vi "输入数据解析.vi"(0 "单个参数补充":dbl, 1 "从板号":dbl=1.0, 2 "主板二维码":string="BNET01", 3 "从板二维码":string="BNET01", 5 "主板引用":refnum<vi>, 7 "从板引用":refnum<vi>, 9 "主板选项":string="三级故障阀值", 11 "枚举":enum16{"主板", "从板"}(ring), 12 "快换":bool caption="快换写入") -> (4 "输出数组":dbl[][](array[numeric]), 6 "数组长度":dbl[](array[numeric]), 8 "循环次数":i32, 10 "命令":u32, 14 "名称":string[](array[string]), 15 "命令序号":u32[](array[numeric]))   [LabVIEW 2013] (continued)
              tunnel: [w13384 w13395 w13406 w13418 w13429 w13440 w13452 w13462] -> w13379
              frame 0, Default {
                # "最大允许单体电压"
                n5117 = disable-structure shown="启用" {
                  disable-tunnel: [w13390 w13393] -> w13386
                  disable-tunnel: [w13389 w13393] -> w13385
                  disable-tunnel: w13383 -> [w13388 _]
                  frame Disabled {
                    n5118 = Unbundle By Name(w13388) -> ("最大允许单体电压"=w13387:dbl)
                    n5119 = call "输入分辨率计算-EV05.vi"("1字节?"=FALSE, "数值"=w13387, "分辨率"=0.001) -> ("低字节"=w13389:dbl, "高字节1"=w13390:dbl)  [unwired: 2 in, 5 out]
                  }
                  frame Enabled {
                    w13393 = 255 ("高字节1")
                  }
                }
                n5120 = Build Array(w13386, w13385) -> (w13384:i32[])
              }
              frame 1 {
                # "最大允许总电压"
                n5121 = disable-structure shown="启用" {
                  disable-tunnel: [w13401 w13404] -> w13397
                  disable-tunnel: [w13400 w13404] -> w13396
                  disable-tunnel: w13394 -> [w13399 _]
                  frame Disabled {
                    n5122 = Unbundle By Name(w13399) -> ("最大允许总电压"=w13398:dbl)
                    n5123 = call "输入分辨率计算-EV05.vi"("1字节?"=FALSE, "数值"=w13398, "分辨率"=0.1) -> ("低字节"=w13400:dbl, "高字节1"=w13401:dbl)  [unwired: 2 in, 5 out]
                  }
                  frame Enabled {
                    w13404 = 255 ("高字节1")
                  }
                }
                n5124 = Build Array(w13397, w13396) -> (w13395:i32[])
              }
              frame 2 {
                # "最大允许充电电流"
                n5125 = disable-structure shown="启用" {
                  disable-tunnel: [w13413 w13416] -> w13408
                  disable-tunnel: [w13412 w13416] -> w13407
                  disable-tunnel: w13405 -> [w13410 _]
                  frame Enabled {
                    n5126 = Unbundle By Name(w13410) -> ("最大允许充电电流"=w13409:dbl)
                    n5127 = call "输入分辨率计算-EV05.vi"("1字节?"=FALSE, "数值"=w13409, "偏移量"=0.0, "分辨率"=0.1) -> ("低字节"=w13412:dbl, "高字节1"=w13413:dbl)  [unwired: 1 in, 5 out]
                  }
                  frame Disabled {
                    w13416 = 255 ("高字节1")
                  }
                }
                n5128 = Build Array(w13408, w13407) -> (w13406:dbl[])
              }
              frame 3 {
                # "最小允许充电温度"
                n5129 = disable-structure shown="启用" {
                  disable-tunnel: [w13423 255 ("高字节1")] -> w13419
                  disable-tunnel: w13417 -> [w13421 _]
                  frame Disabled {
                    n5130 = Unbundle By Name(w13421) -> ("最小允许温度"=w13420:dbl)
                    n5131 = call "输入分辨率计算-EV05.vi"("1字节?"=TRUE, "数值"=w13420, "偏移量"=-40.0, "分辨率"=1.0) -> ("高字节1"=w13423:dbl)  [unwired: 1 in, 6 out]
                  }
                  frame Enabled {
                  }
                }
                n5132 = Build Array(w13419) -> (w13418:i32[])
              }
              frame 4 {
                # "最小充电电流"
                n5133 = disable-structure shown="启用" {
                  disable-tunnel: [w13434 w13437] -> w13430
                  disable-tunnel: [w13433 w13437] -> w13428
                  disable-tunnel: w13427 -> [w13432 _]
                  frame Disabled {
                    n5134 = Unbundle By Name(w13432) -> ("最小充电电流"=w13431:dbl)
                    n5135 = call "输入分辨率计算-EV05.vi"("1字节?"=FALSE, "数值"=w13431, "分辨率"=0.1) -> ("低字节"=w13433:dbl, "高字节1"=w13434:dbl)  [unwired: 2 in, 5 out]
                  }
                  frame Enabled {
                    w13437 = 255 ("高字节1")
                  }
                }
                n5136 = Build Array(w13430, w13428) -> (w13429:i32[])
              }
              frame 5 {
                # "电流步长"
                n5137 = disable-structure shown="启用" {
                  disable-tunnel: [w13446 w13449] -> w13441
                  disable-tunnel: [w13444 w13449] -> w13439
                  disable-tunnel: w13438 -> [w13443 _]
                  frame Disabled {
                    n5138 = Unbundle By Name(w13443) -> ("电流步长"=w13442:dbl)
                    n5139 = call "输入分辨率计算-EV05.vi"("1字节?"=FALSE, "数值"=w13442, "偏移量"=0.0, "分辨率"=1.0) -> ("低字节"=w13444:dbl, "高字节1"=w13446:dbl)  [unwired: 1 in, 5 out]
                  }
                  frame Enabled {
                    w13449 = 255 ("高字节1")
                  }
                }
                n5140 = Build Array(w13441, w13439) -> (w13440:i32[])
              }
              frame 6 {
                # "最小允许单体电压"
                n5141 = disable-structure shown="启用" {
                  disable-tunnel: [w13457 w13460] -> w13453
                  disable-tunnel: [w13456 w13460] -> w13451
                  disable-tunnel: w13450 -> [w13455 _]
                  frame Disabled {
                    n5142 = Unbundle By Name(w13455) -> ("最小允许单体电压"=w13454:dbl)
                    n5143 = call "输入分辨率计算-EV05.vi"("1字节?"=FALSE, "数值"=w13454, "分辨率"=0.001) -> ("低字节"=w13456:dbl, "高字节1"=w13457:dbl)  [unwired: 2 in, 5 out]
                  }
                  frame Enabled {
                    w13460 = 255 ("高字节1")
                  }
                }
                n5144 = Build Array(w13453, w13451) -> (w13452:i32[])
              }
              frame 7 {
                # "最大允许充电温度"
                n5145 = disable-structure shown="启用" {
                  disable-tunnel: [w13467 255 ("高字节1")] -> w13463
                  disable-tunnel: w13461 -> [w13465 _]
                  frame Disabled {
                    n5146 = Unbundle By Name(w13465) -> ("最大允许充电温度"=w13464:dbl)
                    n5147 = call "输入分辨率计算-EV05.vi"("1字节?"=TRUE, "数值"=w13464, "偏移量"=-40.0, "分辨率"=1.0) -> ("高字节1"=w13467:dbl)  [unwired: 1 in, 6 out]
                  }
                  frame Enabled {
                  }
                }
                n5148 = Build Array(w13463) -> (w13462:i32[])
              }
            }
            n5149 = Insert Into Array(array=w13378, new element=w13379) -> (w13382:dbl[])  [unwired: 1 in]
          }
          n5150 = Build Array(w13374) -> (w13376:dbl[][])
        }
        frame "最小允许充电温度" {
          n5151 = Unbundle By Name(w13474) -> ("充电控制参数"=w13475:refnum<vi>)
          n5152 = property class="Clust (严格)"(reference=w13475) -> ("Value"=w13473:T6)  [unwired: 1 in, 2 out]
          n5153 = for {
            N: 8 -> [_]
            tunnel: w13473 -> [w13485]
            shift-right: [w13487] -> w13479
            shift-left: dbl[] [] -> [w13483]
            i -> [w13486]
            n5154 = case shown="3" w13486 {
              tunnel: w13485 -> [w13488 w13499 w13510 w13522 w13532 w13543 w13555 w13566]
              tunnel: [w13489 w13500 w13511 w13523 w13534 w13545 w13557 w13567] -> w13484
              frame 0, Default {
                # "最大允许单体电压"
                n5155 = disable-structure shown="启用" {
                  disable-tunnel: [w13495 w13498] -> w13491
                  disable-tunnel: [w13494 w13498] -> w13490
                  disable-tunnel: w13488 -> [w13493 _]
                  frame Disabled {
                    n5156 = Unbundle By Name(w13493) -> ("最大允许单体电压"=w13492:dbl)
                    n5157 = call "输入分辨率计算-EV05.vi"("1字节?"=FALSE, "数值"=w13492, "分辨率"=0.001) -> ("低字节"=w13494:dbl, "高字节1"=w13495:dbl)  [unwired: 2 in, 5 out]
                  }
                  frame Enabled {
                    w13498 = 255 ("高字节1")
                  }
                }
                n5158 = Build Array(w13491, w13490) -> (w13489:i32[])
              }
              frame 1 {
                # "最大允许总电压"
                n5159 = disable-structure shown="启用" {
                  disable-tunnel: [w13506 w13509] -> w13502
                  disable-tunnel: [w13505 w13509] -> w13501
                  disable-tunnel: w13499 -> [w13504 _]
                  frame Disabled {
                    n5160 = Unbundle By Name(w13504) -> ("最大允许总电压"=w13503:dbl)
                    n5161 = call "输入分辨率计算-EV05.vi"("1字节?"=FALSE, "数值"=w13503, "分辨率"=0.1) -> ("低字节"=w13505:dbl, "高字节1"=w13506:dbl)  [unwired: 2 in, 5 out]
                  }
                  frame Enabled {
                    w13509 = 255 ("高字节1")
                  }
                }
                n5162 = Build Array(w13502, w13501) -> (w13500:i32[])
              }
              frame 2 {
                # "最大允许充电电流"
                n5163 = disable-structure shown="启用" {
                  disable-tunnel: [w13518 w13521] -> w13513
                  disable-tunnel: [w13517 w13521] -> w13512
                  disable-tunnel: w13510 -> [w13515 _]
                  frame Disabled {
                    n5164 = Unbundle By Name(w13515) -> ("最大允许充电电流"=w13514:dbl)
                    n5165 = call "输入分辨率计算-EV05.vi"("1字节?"=FALSE, "数值"=w13514, "偏移量"=-3000.0, "分辨率"=0.1) -> ("低字节"=w13517:dbl, "高字节1"=w13518:dbl)  [unwired: 1 in, 5 out]
                  }
                  frame Enabled {
                    w13521 = 255 ("高字节1")
                  }
                }
                n5166 = Build Array(w13513, w13512) -> (w13511:i32[])
              }
              frame 3 {
                # "最小允许充电温度"
                n5167 = disable-structure shown="启用" {
                  disable-tunnel: [w13528 255 ("高字节1")] -> w13524
                  disable-tunnel: w13522 -> [w13526 _]
                  frame Enabled {
                    n5168 = Unbundle By Name(w13526) -> ("最小允许充电温度"=w13525:dbl)
                    n5169 = call "输入分辨率计算-EV05.vi"("1字节?"=TRUE, "数值"=w13525, "偏移量"=-40.0, "分辨率"=1.0) -> ("高字节1"=w13528:dbl)  [unwired: 1 in, 6 out]
                  }
                  frame Disabled {
                  }
                }
                n5170 = Build Array(w13524) -> (w13523:dbl[])
              }
              frame 4 {
                # "最小充电电流"
                n5171 = disable-structure shown="启用" {
                  disable-tunnel: [w13539 w13542] -> w13535
                  disable-tunnel: [w13538 w13542] -> w13533
                  disable-tunnel: w13532 -> [w13537 _]
                  frame Disabled {
                    n5172 = Unbundle By Name(w13537) -> ("最小充电电流"=w13536:dbl)
                    n5173 = call "输入分辨率计算-EV05.vi"("1字节?"=FALSE, "数值"=w13536, "分辨率"=0.1) -> ("低字节"=w13538:dbl, "高字节1"=w13539:dbl)  [unwired: 2 in, 5 out]
                  }
                  frame Enabled {
                    w13542 = 255 ("高字节1")
                  }
                }
                n5174 = Build Array(w13535, w13533) -> (w13534:i32[])
              }
              frame 5 {
                # "电流步长"
                n5175 = disable-structure shown="启用" {
                  disable-tunnel: [w13551 w13554] -> w13546
                  disable-tunnel: [w13549 w13554] -> w13544
                  disable-tunnel: w13543 -> [w13548 _]
                  frame Disabled {
                    n5176 = Unbundle By Name(w13548) -> ("电流步长"=w13547:dbl)
                    n5177 = call "输入分辨率计算-EV05.vi"("1字节?"=FALSE, "数值"=w13547, "偏移量"=0.0, "分辨率"=1.0) -> ("低字节"=w13549:dbl, "高字节1"=w13551:dbl)  [unwired: 1 in, 5 out]
                  }
                  frame Enabled {
                    w13554 = 255 ("高字节1")
                  }
                }
                n5178 = Build Array(w13546, w13544) -> (w13545:i32[])
              }
              frame 6 {
                # "最小允许单体电压"
                n5179 = disable-structure shown="启用" {
                  disable-tunnel: [w13562 w13565] -> w13558
                  disable-tunnel: [w13561 w13565] -> w13556
                  disable-tunnel: w13555 -> [w13560 _]
                  frame Disabled {
                    n5180 = Unbundle By Name(w13560) -> ("最小允许单体电压"=w13559:dbl)
                    n5181 = call "输入分辨率计算-EV05.vi"("1字节?"=FALSE, "数值"=w13559, "分辨率"=0.001) -> ("低字节"=w13561:dbl, "高字节1"=w13562:dbl)  [unwired: 2 in, 5 out]
                  }
                  frame Enabled {
                    w13565 = 255 ("高字节1")
                  }
                }
                n5182 = Build Array(w13558, w13556) -> (w13557:i32[])
              }
              frame 7 {
                # "最大允许充电温度"
                n5183 = disable-structure shown="启用" {
                  disable-tunnel: [w13572 255 ("高字节1")] -> w13568
                  disable-tunnel: w13566 -> [w13570 _]
                  frame Disabled {
                    n5184 = Unbundle By Name(w13570) -> ("最大允许充电温度"=w13569:dbl)
                    n5185 = call "输入分辨率计算-EV05.vi"("1字节?"=TRUE, "数值"=w13569, "偏移量"=-40.0, "分辨率"=1.0) -> ("高字节1"=w13572:dbl)  [unwired: 1 in, 6 out]
                  }
                  frame Enabled {
                  }
                }
                n5186 = Build Array(w13568) -> (w13567:i32[])
              }
            }
            n5187 = Insert Into Array(array=w13483, new element=w13484) -> (w13487:dbl[])  [unwired: 1 in]
          }
          n5188 = Build Array(w13479) -> (w13481:dbl[][])
        }
        frame "最小允许充电电流" {
          n5189 = Unbundle By Name(w13579) -> ("充电控制参数"=w13580:refnum<vi>)
          n5190 = property class="Clust (严格)"(reference=w13580) -> ("Value"=w13578:T6)  [unwired: 1 in, 2 out]
          n5191 = for {
            N: 8 -> [_]
            tunnel: w13578 -> [w13590]
            shift-right: [w13592] -> w13584
            shift-left: dbl[] [] -> [w13588]
            i -> [w13591]
            n5192 = case shown="4" w13591 {
              tunnel: w13590 -> [w13593 w13604 w13615 w13627 w13637 w13648 w13660 w13671]
              tunnel: [w13594 w13605 w13616 w13628 w13639 w13650 w13662 w13672] -> w13589
              frame 0, Default {
                # "最大允许单体电压"
                n5193 = disable-structure shown="启用" {
                  disable-tunnel: [w13600 w13603] -> w13596
                  disable-tunnel: [w13599 w13603] -> w13595
                  disable-tunnel: w13593 -> [w13598 _]
                  frame Disabled {
                    n5194 = Unbundle By Name(w13598) -> ("最大允许单体电压"=w13597:dbl)
                    n5195 = call "输入分辨率计算-EV05.vi"("1字节?"=FALSE, "数值"=w13597, "分辨率"=0.001) -> ("低字节"=w13599:dbl, "高字节1"=w13600:dbl)  [unwired: 2 in, 5 out]
                  }
                  frame Enabled {
                    w13603 = 255 ("高字节1")
                  }
                }
                n5196 = Build Array(w13596, w13595) -> (w13594:i32[])
              }
              frame 1 {
                # "最大允许总电压"
                n5197 = disable-structure shown="启用" {
                  disable-tunnel: [w13611 w13614] -> w13607
                  disable-tunnel: [w13610 w13614] -> w13606
                  disable-tunnel: w13604 -> [w13609 _]
                  frame Disabled {
                    n5198 = Unbundle By Name(w13609) -> ("最大允许总电压"=w13608:dbl)
                    n5199 = call "输入分辨率计算-EV05.vi"("1字节?"=FALSE, "数值"=w13608, "分辨率"=0.1) -> ("低字节"=w13610:dbl, "高字节1"=w13611:dbl)  [unwired: 2 in, 5 out]
                  }
                  frame Enabled {
                    w13614 = 255 ("高字节1")
                  }
                }
                n5200 = Build Array(w13607, w13606) -> (w13605:i32[])
              }
              frame 2 {
                # "最大允许充电电流"
                n5201 = disable-structure shown="启用" {
                  disable-tunnel: [w13623 w13626] -> w13618
                  disable-tunnel: [w13622 w13626] -> w13617
                  disable-tunnel: w13615 -> [w13620 _]
                  frame Disabled {
                    n5202 = Unbundle By Name(w13620) -> ("最大允许充电电流"=w13619:dbl)
                    n5203 = call "输入分辨率计算-EV05.vi"("1字节?"=FALSE, "数值"=w13619, "偏移量"=-3000.0, "分辨率"=0.1) -> ("低字节"=w13622:dbl, "高字节1"=w13623:dbl)  [unwired: 1 in, 5 out]
                  }
                  frame Enabled {
                    w13626 = 255 ("高字节1")
                  }
                }
                n5204 = Build Array(w13618, w13617) -> (w13616:i32[])
              }
              frame 3 {
                # "最小允许充电温度"
                n5205 = disable-structure shown="启用" {
                  disable-tunnel: [w13633 255 ("高字节1")] -> w13629
                  disable-tunnel: w13627 -> [w13631 _]
                  frame Disabled {
                    n5206 = Unbundle By Name(w13631) -> ("最小允许温度"=w13630:dbl)
                    n5207 = call "输入分辨率计算-EV05.vi"("1字节?"=TRUE, "数值"=w13630, "偏移量"=-40.0, "分辨率"=1.0) -> ("高字节1"=w13633:dbl)  [unwired: 1 in, 6 out]
                  }
                  frame Enabled {
                  }
                }
                n5208 = Build Array(w13629) -> (w13628:i32[])
              }
              frame 4 {
                # "最小充电电流"
                n5209 = disable-structure shown="启用" {
                  disable-tunnel: [w13644 w13647] -> w13640
                  disable-tunnel: [w13643 w13647] -> w13638
                  disable-tunnel: w13637 -> [w13642 _]
                  frame Enabled {
                    n5210 = Unbundle By Name(w13642) -> ("最小允许充电电流"=w13641:dbl)
                    n5211 = call "输入分辨率计算-EV05.vi"("1字节?"=FALSE, "数值"=w13641, "分辨率"=0.1) -> ("低字节"=w13643:dbl, "高字节1"=w13644:dbl)  [unwired: 2 in, 5 out]
                  }
                  frame Disabled {
                    w13647 = 255 ("高字节1")
                  }
                }
                n5212 = Build Array(w13640, w13638) -> (w13639:dbl[])
              }
              frame 5 {
                # "电流步长"
                n5213 = disable-structure shown="启用" {
                  disable-tunnel: [w13656 w13659] -> w13651
                  disable-tunnel: [w13654 w13659] -> w13649
                  disable-tunnel: w13648 -> [w13653 _]
                  frame Disabled {
                    n5214 = Unbundle By Name(w13653) -> ("电流步长"=w13652:dbl)
                    n5215 = call "输入分辨率计算-EV05.vi"("1字节?"=FALSE, "数值"=w13652, "偏移量"=0.0, "分辨率"=1.0) -> ("低字节"=w13654:dbl, "高字节1"=w13656:dbl)  [unwired: 1 in, 5 out]
                  }
                  frame Enabled {
                    w13659 = 255 ("高字节1")
                  }
                }
                n5216 = Build Array(w13651, w13649) -> (w13650:i32[])
              }
              frame 6 {
                # "最小允许单体电压"
                n5217 = disable-structure shown="启用" {
                  disable-tunnel: [w13667 w13670] -> w13663
                  disable-tunnel: [w13666 w13670] -> w13661
                  disable-tunnel: w13660 -> [w13665 _]
                  frame Disabled {
                    n5218 = Unbundle By Name(w13665) -> ("最小允许单体电压"=w13664:dbl)
                    n5219 = call "输入分辨率计算-EV05.vi"("1字节?"=FALSE, "数值"=w13664, "分辨率"=0.001) -> ("低字节"=w13666:dbl, "高字节1"=w13667:dbl)  [unwired: 2 in, 5 out]
                  }
                  frame Enabled {
                    w13670 = 255 ("高字节1")
                  }
                }
                n5220 = Build Array(w13663, w13661) -> (w13662:i32[])
              }
              frame 7 {
                # "最大允许充电温度"
                n5221 = disable-structure shown="启用" {
                  disable-tunnel: [w13677 255 ("高字节1")] -> w13673
                  disable-tunnel: w13671 -> [w13675 _]
                  frame Disabled {
                    n5222 = Unbundle By Name(w13675) -> ("最大允许充电温度"=w13674:dbl)
                    n5223 = call "输入分辨率计算-EV05.vi"("1字节?"=TRUE, "数值"=w13674, "偏移量"=-40.0, "分辨率"=1.0) -> ("高字节1"=w13677:dbl)  [unwired: 1 in, 6 out]
                  }
                  frame Enabled {
                  }
                }
                n5224 = Build Array(w13673) -> (w13672:i32[])
              }
            }
            n5225 = Insert Into Array(array=w13588, new element=w13589) -> (w13592:dbl[])  [unwired: 1 in]
          }
          n5226 = Build Array(w13584) -> (w13586:dbl[][])
        }
        frame "电流步长" {
          n5227 = Unbundle By Name(w13684) -> ("充电控制参数"=w13685:refnum<vi>)
          n5228 = property class="Clust (严格)"(reference=w13685) -> ("Value"=w13683:T6)  [unwired: 1 in, 2 out]
          n5229 = for {
            N: 8 -> [_]
            tunnel: w13683 -> [w13695]
            shift-right: [w13697] -> w13689
            shift-left: dbl[] [] -> [w13693]
            i -> [w13696]
            n5230 = case shown="5" w13696 {
              tunnel: w13695 -> [w13698 w13709 w13720 w13732 w13742 w13753 w13765 w13776]
              tunnel: [w13699 w13710 w13721 w13733 w13744 w13755 w13767 w13777] -> w13694
              frame 0, Default {
                # "最大允许单体电压"
                n5231 = disable-structure shown="启用" {
                  disable-tunnel: [w13705 w13708] -> w13701
                  disable-tunnel: [w13704 w13708] -> w13700
                  disable-tunnel: w13698 -> [w13703 _]
                  frame Disabled {
                    n5232 = Unbundle By Name(w13703) -> ("最大允许单体电压"=w13702:dbl)
                    n5233 = call "输入分辨率计算-EV05.vi"("1字节?"=FALSE, "数值"=w13702, "分辨率"=0.001) -> ("低字节"=w13704:dbl, "高字节1"=w13705:dbl)  [unwired: 2 in, 5 out]
                  }
                  frame Enabled {
                    w13708 = 255 ("高字节1")
                  }
                }
                n5234 = Build Array(w13701, w13700) -> (w13699:i32[])
              }
              frame 1 {
                # "最大允许总电压"
                n5235 = disable-structure shown="启用" {
                  disable-tunnel: [w13716 w13719] -> w13712
                  disable-tunnel: [w13715 w13719] -> w13711
                  disable-tunnel: w13709 -> [w13714 _]
                  frame Disabled {
                    n5236 = Unbundle By Name(w13714) -> ("最大允许总电压"=w13713:dbl)
                    n5237 = call "输入分辨率计算-EV05.vi"("1字节?"=FALSE, "数值"=w13713, "分辨率"=0.1) -> ("低字节"=w13715:dbl, "高字节1"=w13716:dbl)  [unwired: 2 in, 5 out]
                  }
                  frame Enabled {
                    w13719 = 255 ("高字节1")
                  }
                }
                n5238 = Build Array(w13712, w13711) -> (w13710:i32[])
              }
              frame 2 {
                # "最大允许充电电流"
                n5239 = disable-structure shown="启用" {
                  disable-tunnel: [w13728 w13731] -> w13723
                  disable-tunnel: [w13727 w13731] -> w13722
                  disable-tunnel: w13720 -> [w13725 _]
                  frame Disabled {
                    n5240 = Unbundle By Name(w13725) -> ("最大允许充电电流"=w13724:dbl)
                    n5241 = call "输入分辨率计算-EV05.vi"("1字节?"=FALSE, "数值"=w13724, "偏移量"=-3000.0, "分辨率"=0.1) -> ("低字节"=w13727:dbl, "高字节1"=w13728:dbl)  [unwired: 1 in, 5 out]
                  }
                  frame Enabled {
                    w13731 = 255 ("高字节1")
                  }
                }
                n5242 = Build Array(w13723, w13722) -> (w13721:i32[])
              }
              frame 3 {
                # "最小允许充电温度"
                n5243 = disable-structure shown="启用" {
                  disable-tunnel: [w13738 255 ("高字节1")] -> w13734
                  disable-tunnel: w13732 -> [w13736 _]
                  frame Disabled {
                    n5244 = Unbundle By Name(w13736) -> ("最小允许温度"=w13735:dbl)
                    n5245 = call "输入分辨率计算-EV05.vi"("1字节?"=TRUE, "数值"=w13735, "偏移量"=-40.0, "分辨率"=1.0) -> ("高字节1"=w13738:dbl)  [unwired: 1 in, 6 out]
                  }
                  frame Enabled {
                  }
                }
                n5246 = Build Array(w13734) -> (w13733:i32[])
              }
              frame 4 {
                # "最小充电电流"
                n5247 = disable-structure shown="启用" {
                  disable-tunnel: [w13749 w13752] -> w13745
                  disable-tunnel: [w13748 w13752] -> w13743
                  disable-tunnel: w13742 -> [w13747 _]
                  frame Disabled {
                    n5248 = Unbundle By Name(w13747) -> ("最小充电电流"=w13746:dbl)
                    n5249 = call "输入分辨率计算-EV05.vi"("1字节?"=FALSE, "数值"=w13746, "分辨率"=0.1) -> ("低字节"=w13748:dbl, "高字节1"=w13749:dbl)  [unwired: 2 in, 5 out]
                  }
                  frame Enabled {
                    w13752 = 255 ("高字节1")
                  }
                }
                n5250 = Build Array(w13745, w13743) -> (w13744:i32[])
              }
              frame 5 {
                # "电流步长"
                n5251 = disable-structure shown="启用" {
                  disable-tunnel: [w13761 w13764] -> w13756
                  disable-tunnel: [w13759 w13764] -> w13754
                  disable-tunnel: w13753 -> [w13758 _]
                  frame Enabled {
                    n5252 = Unbundle By Name(w13758) -> ("电流步长"=w13757:dbl)
                    n5253 = call "输入分辨率计算-EV05.vi"("1字节?"=FALSE, "数值"=w13757, "偏移量"=0.0, "分辨率"=0.1) -> ("低字节"=w13759:dbl, "高字节1"=w13761:dbl)  [unwired: 1 in, 5 out]
                  }
                  frame Disabled {
                    w13764 = 255 ("高字节1")
                  }
                }
                n5254 = Build Array(w13756, w13754) -> (w13755:dbl[])
              }
              frame 6 {
                # "最小允许单体电压"
                n5255 = disable-structure shown="启用" {
                  disable-tunnel: [w13772 w13775] -> w13768
                  disable-tunnel: [w13771 w13775] -> w13766
                  disable-tunnel: w13765 -> [w13770 _]
                  frame Disabled {
                    n5256 = Unbundle By Name(w13770) -> ("最小允许单体电压"=w13769:dbl)
                    n5257 = call "输入分辨率计算-EV05.vi"("1字节?"=FALSE, "数值"=w13769, "分辨率"=0.001) -> ("低字节"=w13771:dbl, "高字节1"=w13772:dbl)  [unwired: 2 in, 5 out]
                  }
                  frame Enabled {
                    w13775 = 255 ("高字节1")
                  }
                }
                n5258 = Build Array(w13768, w13766) -> (w13767:i32[])
              }
              frame 7 {
                # "最大允许充电温度"
                n5259 = disable-structure shown="启用" {
                  disable-tunnel: [w13782 255 ("高字节1")] -> w13778
                  disable-tunnel: w13776 -> [w13780 _]
                  frame Disabled {
                    n5260 = Unbundle By Name(w13780) -> ("最大允许充电温度"=w13779:dbl)
                    n5261 = call "输入分辨率计算-EV05.vi"("1字节?"=TRUE, "数值"=w13779, "偏移量"=-40.0, "分辨率"=1.0) -> ("高字节1"=w13782:dbl)  [unwired: 1 in, 6 out]
                  }
                  frame Enabled {
                  }
                }
                n5262 = Build Array(w13778) -> (w13777:i32[])
              }
            }
            n5263 = Insert Into Array(array=w13693, new element=w13694) -> (w13697:dbl[])  [unwired: 1 in]
          }
          n5264 = Build Array(w13689) -> (w13691:dbl[][])
        }
        frame "最小允许单体电压" {
          n5265 = Unbundle By Name(w13789) -> ("充电控制参数"=w13790:refnum<vi>)
          n5266 = property class="Clust (严格)"(reference=w13790) -> ("Value"=w13788:T6)  [unwired: 1 in, 2 out]
          n5267 = for {
            N: 8 -> [_]
            tunnel: w13788 -> [w13800]
            shift-right: [w13802] -> w13794
            shift-left: dbl[] [] -> [w13798]
            i -> [w13801]
            n5268 = case shown="6" w13801 {
              tunnel: w13800 -> [w13803 w13814 w13825 w13837 w13847 w13858 w13870 w13881]
              tunnel: [w13804 w13815 w13826 w13838 w13849 w13860 w13872 w13882] -> w13799
              frame 0, Default {
                # "最大允许单体电压"
                n5269 = disable-structure shown="启用" {
                  disable-tunnel: [w13810 w13813] -> w13806
                  disable-tunnel: [w13809 w13813] -> w13805
                  disable-tunnel: w13803 -> [w13808 _]
                  frame Disabled {
                    n5270 = Unbundle By Name(w13808) -> ("最大允许单体电压"=w13807:dbl)
                    n5271 = call "输入分辨率计算-EV05.vi"("1字节?"=FALSE, "数值"=w13807, "分辨率"=0.001) -> ("低字节"=w13809:dbl, "高字节1"=w13810:dbl)  [unwired: 2 in, 5 out]
                  }
                  frame Enabled {
                    w13813 = 255 ("高字节1")
                  }
                }
                n5272 = Build Array(w13806, w13805) -> (w13804:i32[])
              }
              frame 1 {
                # "最大允许总电压"
                n5273 = disable-structure shown="启用" {
                  disable-tunnel: [w13821 w13824] -> w13817
                  disable-tunnel: [w13820 w13824] -> w13816
                  disable-tunnel: w13814 -> [w13819 _]
                  frame Disabled {
                    n5274 = Unbundle By Name(w13819) -> ("最大允许总电压"=w13818:dbl)
                    n5275 = call "输入分辨率计算-EV05.vi"("1字节?"=FALSE, "数值"=w13818, "分辨率"=0.1) -> ("低字节"=w13820:dbl, "高字节1"=w13821:dbl)  [unwired: 2 in, 5 out]
                  }
                  frame Enabled {
                    w13824 = 255 ("高字节1")
                  }
                }
                n5276 = Build Array(w13817, w13816) -> (w13815:i32[])
              }
              frame 2 {
                # "最大允许充电电流"
                n5277 = disable-structure shown="启用" {
                  disable-tunnel: [w13833 w13836] -> w13828
                  disable-tunnel: [w13832 w13836] -> w13827
                  disable-tunnel: w13825 -> [w13830 _]
                  frame Disabled {
                    n5278 = Unbundle By Name(w13830) -> ("最大允许充电电流"=w13829:dbl)
                    n5279 = call "输入分辨率计算-EV05.vi"("1字节?"=FALSE, "数值"=w13829, "偏移量"=-3000.0, "分辨率"=0.1) -> ("低字节"=w13832:dbl, "高字节1"=w13833:dbl)  [unwired: 1 in, 5 out]
                  }
                  frame Enabled {
                    w13836 = 255 ("高字节1")
                  }
                }
                n5280 = Build Array(w13828, w13827) -> (w13826:i32[])
              }
              frame 3 {
                # "最小允许充电温度"
                n5281 = disable-structure shown="启用" {
                  disable-tunnel: [w13843 255 ("高字节1")] -> w13839
                  disable-tunnel: w13837 -> [w13841 _]
                  frame Disabled {
                    n5282 = Unbundle By Name(w13841) -> ("最小允许温度"=w13840:dbl)
                    n5283 = call "输入分辨率计算-EV05.vi"("1字节?"=TRUE, "数值"=w13840, "偏移量"=-40.0, "分辨率"=1.0) -> ("高字节1"=w13843:dbl)  [unwired: 1 in, 6 out]
                  }
                  frame Enabled {
                  }
                }
                n5284 = Build Array(w13839) -> (w13838:i32[])
              }
              frame 4 {
                # "最小充电电流"
                n5285 = disable-structure shown="启用" {
                  disable-tunnel: [w13854 w13857] -> w13850
                  disable-tunnel: [w13853 w13857] -> w13848
                  disable-tunnel: w13847 -> [w13852 _]
                  frame Disabled {
                    n5286 = Unbundle By Name(w13852) -> ("最小充电电流"=w13851:dbl)
                    n5287 = call "输入分辨率计算-EV05.vi"("1字节?"=FALSE, "数值"=w13851, "分辨率"=0.1) -> ("低字节"=w13853:dbl, "高字节1"=w13854:dbl)  [unwired: 2 in, 5 out]
                  }
                  frame Enabled {
                    w13857 = 255 ("高字节1")
                  }
                }
                n5288 = Build Array(w13850, w13848) -> (w13849:i32[])
              }
              frame 5 {
                # "电流步长"
                n5289 = disable-structure shown="启用" {
                  disable-tunnel: [w13866 w13869] -> w13861
                  disable-tunnel: [w13864 w13869] -> w13859
                  disable-tunnel: w13858 -> [w13863 _]
                  frame Disabled {
                    n5290 = Unbundle By Name(w13863) -> ("电流步长"=w13862:dbl)
                    n5291 = call "输入分辨率计算-EV05.vi"("1字节?"=FALSE, "数值"=w13862, "偏移量"=0.0, "分辨率"=1.0) -> ("低字节"=w13864:dbl, "高字节1"=w13866:dbl)  [unwired: 1 in, 5 out]
                  }
                  frame Enabled {
                    w13869 = 255 ("高字节1")
                  }
                }
                n5292 = Build Array(w13861, w13859) -> (w13860:i32[])
              }
              frame 6 {
                # "最小允许单体电压"
                n5293 = disable-structure shown="启用" {
                  disable-tunnel: [w13877 w13880] -> w13873
                  disable-tunnel: [w13876 w13880] -> w13871
                  disable-tunnel: w13870 -> [w13875 _]
                  frame Enabled {
                    n5294 = Unbundle By Name(w13875) -> ("最小允许单体电压"=w13874:dbl)
                    n5295 = call "输入分辨率计算-EV05.vi"("1字节?"=FALSE, "数值"=w13874, "分辨率"=0.001) -> ("低字节"=w13876:dbl, "高字节1"=w13877:dbl)  [unwired: 2 in, 5 out]
                  }
                  frame Disabled {
                    w13880 = 255 ("高字节1")
                  }
                }
                n5296 = Build Array(w13873, w13871) -> (w13872:dbl[])
              }
              frame 7 {
                # "最大允许充电温度"
                n5297 = disable-structure shown="启用" {
                  disable-tunnel: [w13887 255 ("高字节1")] -> w13883
                  disable-tunnel: w13881 -> [w13885 _]
                  frame Disabled {
                    n5298 = Unbundle By Name(w13885) -> ("最大允许充电温度"=w13884:dbl)
                    n5299 = call "输入分辨率计算-EV05.vi"("1字节?"=TRUE, "数值"=w13884, "偏移量"=-40.0, "分辨率"=1.0) -> ("高字节1"=w13887:dbl)  [unwired: 1 in, 6 out]
                  }
                  frame Enabled {
                  }
                }
                n5300 = Build Array(w13883) -> (w13882:i32[])
              }
            }
            n5301 = Insert Into Array(array=w13798, new element=w13799) -> (w13802:dbl[])  [unwired: 1 in]
          }
          n5302 = Build Array(w13794) -> (w13796:dbl[][])
        }
        frame "最大允许充电温度" {
          n5303 = Unbundle By Name(w13894) -> ("充电控制参数"=w13895:refnum<vi>)
          n5304 = property class="Clust (严格)"(reference=w13895) -> ("Value"=w13893:T6)  [unwired: 1 in, 2 out]
          n5305 = for {
            N: 8 -> [_]
            tunnel: w13893 -> [w13905]
            shift-right: [w13907] -> w13899
            shift-left: dbl[] [] -> [w13903]
            i -> [w13906]
            n5306 = case shown="7" w13906 {
              tunnel: w13905 -> [w13908 w13919 w13930 w13942 w13952 w13963 w13975 w13986]
              tunnel: [w13909 w13920 w13931 w13943 w13954 w13965 w13977 w13987] -> w13904
              frame 0, Default {
                # "最大允许单体电压"
                n5307 = disable-structure shown="启用" {
                  disable-tunnel: [w13915 w13918] -> w13911
                  disable-tunnel: [w13914 w13918] -> w13910
                  disable-tunnel: w13908 -> [w13913 _]
                  frame Disabled {
                    n5308 = Unbundle By Name(w13913) -> ("最大允许单体电压"=w13912:dbl)
                    n5309 = call "输入分辨率计算-EV05.vi"("1字节?"=FALSE, "数值"=w13912, "分辨率"=0.001) -> ("低字节"=w13914:dbl, "高字节1"=w13915:dbl)  [unwired: 2 in, 5 out]
                  }
                  frame Enabled {
                    w13918 = 255 ("高字节1")
                  }
                }
                n5310 = Build Array(w13911, w13910) -> (w13909:i32[])
              }
              frame 1 {
                # "最大允许总电压"
                n5311 = disable-structure shown="启用" {
                  disable-tunnel: [w13926 w13929] -> w13922
                  disable-tunnel: [w13925 w13929] -> w13921
                  disable-tunnel: w13919 -> [w13924 _]
                  frame Disabled {
                    n5312 = Unbundle By Name(w13924) -> ("最大允许总电压"=w13923:dbl)
                    n5313 = call "输入分辨率计算-EV05.vi"("1字节?"=FALSE, "数值"=w13923, "分辨率"=0.1) -> ("低字节"=w13925:dbl, "高字节1"=w13926:dbl)  [unwired: 2 in, 5 out]
                  }
                  frame Enabled {
                    w13929 = 255 ("高字节1")
                  }
                }
                n5314 = Build Array(w13922, w13921) -> (w13920:i32[])
              }
              frame 2 {
                # "最大允许充电电流"
                n5315 = disable-structure shown="启用" {
                  disable-tunnel: [w13938 w13941] -> w13933
                  disable-tunnel: [w13937 w13941] -> w13932
                  disable-tunnel: w13930 -> [w13935 _]
                  frame Disabled {
                    n5316 = Unbundle By Name(w13935) -> ("最大允许充电电流"=w13934:dbl)
                    n5317 = call "输入分辨率计算-EV05.vi"("1字节?"=FALSE, "数值"=w13934, "偏移量"=-3000.0, "分辨率"=0.1) -> ("低字节"=w13937:dbl, "高字节1"=w13938:dbl)  [unwired: 1 in, 5 out]
                  }
                  frame Enabled {
                    w13941 = 255 ("高字节1")
                  }
                }
                n5318 = Build Array(w13933, w13932) -> (w13931:i32[])
              }
              frame 3 {
                # "最小允许充电温度"
                n5319 = disable-structure shown="启用" {
                  disable-tunnel: [w13948 255 ("高字节1")] -> w13944
                  disable-tunnel: w13942 -> [w13946 _]
                  frame Disabled {
                    n5320 = Unbundle By Name(w13946) -> ("最小允许温度"=w13945:dbl)
                    n5321 = call "输入分辨率计算-EV05.vi"("1字节?"=TRUE, "数值"=w13945, "偏移量"=-40.0, "分辨率"=1.0) -> ("高字节1"=w13948:dbl)  [unwired: 1 in, 6 out]
                  }
                  frame Enabled {
                  }
                }
                n5322 = Build Array(w13944) -> (w13943:i32[])
              }
              frame 4 {
                # "最小充电电流"
                n5323 = disable-structure shown="启用" {
                  disable-tunnel: [w13959 w13962] -> w13955
                  disable-tunnel: [w13958 w13962] -> w13953
                  disable-tunnel: w13952 -> [w13957 _]
                  frame Disabled {
                    n5324 = Unbundle By Name(w13957) -> ("最小充电电流"=w13956:dbl)
                    n5325 = call "输入分辨率计算-EV05.vi"("1字节?"=FALSE, "数值"=w13956, "分辨率"=0.1) -> ("低字节"=w13958:dbl, "高字节1"=w13959:dbl)  [unwired: 2 in, 5 out]
                  }
                  frame Enabled {
                    w13962 = 255 ("高字节1")
                  }
                }
                n5326 = Build Array(w13955, w13953) -> (w13954:i32[])
              }
              frame 5 {
                # "电流步长"
                n5327 = disable-structure shown="启用" {
                  disable-tunnel: [w13971 w13974] -> w13966
                  disable-tunnel: [w13969 w13974] -> w13964
                  disable-tunnel: w13963 -> [w13968 _]
                  frame Disabled {
                    n5328 = Unbundle By Name(w13968) -> ("电流步长"=w13967:dbl)
                    n5329 = call "输入分辨率计算-EV05.vi"("1字节?"=FALSE, "数值"=w13967, "偏移量"=0.0, "分辨率"=1.0) -> ("低字节"=w13969:dbl, "高字节1"=w13971:dbl)  [unwired: 1 in, 5 out]
                  }
                  frame Enabled {
                    w13974 = 255 ("高字节1")
                  }
                }
                n5330 = Build Array(w13966, w13964) -> (w13965:i32[])
              }
              frame 6 {
                # "最小允许单体电压"
                n5331 = disable-structure shown="启用" {
                  disable-tunnel: [w13982 w13985] -> w13978
                  disable-tunnel: [w13981 w13985] -> w13976
                  disable-tunnel: w13975 -> [w13980 _]
                  frame Disabled {
                    n5332 = Unbundle By Name(w13980) -> ("最小允许单体电压"=w13979:dbl)
                    n5333 = call "输入分辨率计算-EV05.vi"("1字节?"=FALSE, "数值"=w13979, "分辨率"=0.001) -> ("低字节"=w13981:dbl, "高字节1"=w13982:dbl)  [unwired: 2 in, 5 out]
                  }
                  frame Enabled {
                    w13985 = 255 ("高字节1")
                  }
                }
                n5334 = Build Array(w13978, w13976) -> (w13977:i32[])
              }
              frame 7 {
                # "最大允许充电温度"
                n5335 = disable-structure shown="启用" {
                  disable-tunnel: [w13992 255 ("高字节1")] -> w13988
                  disable-tunnel: w13986 -> [w13990 _]
                  frame Enabled {
                    n5336 = Unbundle By Name(w13990) -> ("最大允许充电温度"=w13989:dbl)
                    n5337 = call "输入分辨率计算-EV05.vi"("1字节?"=TRUE, "数值"=w13989, "偏移量"=-40.0, "分辨率"=1.0) -> ("高字节1"=w13992:dbl)  [unwired: 1 in, 6 out]
                  }
                  frame Disabled {
                  }
                }
                n5338 = Build Array(w13988) -> (w13987:dbl[])
              }
            }
            n5339 = Insert Into Array(array=w13903, new element=w13904) -> (w13907:dbl[])  [unwired: 1 in]
          }
          n5340 = Build Array(w13899) -> (w13901:dbl[][])
        }
        frame "电池信息1" {
          n5341 = Unbundle By Name(w13999) -> ("电池信息"=w14000:refnum<vi>)
          n5342 = property class="Clust (严格)"(reference=w14000) -> ("Value"=w13998:T7)  [unwired: 1 in, 2 out]
          n5343 = for {
            N: 1 -> [_]
            tunnel: [w14009] -> w14004 mode=indexing
            tunnel: [w14008] -> w14003 mode=indexing
            tunnel: [w14010] -> w14001 mode=indexing
            tunnel: w13998 -> [w14007]
            i -> [w14006]
            n5344 = case shown="0, 默认" w14006 {
              tunnel: [30 ("单个参数补充") 4 ("单个参数补充") 8 ("单个参数补充") 6 ("单个参数补充")] -> w14009
              tunnel: [1 ("命令序号") 2 ("命令序号") 3 ("命令序号") 4 ("命令序号")] -> w14008
              tunnel: [w14059 w14105 w14131 w14143] -> w14010
              tunnel: w14007 -> [w14060 w14104 w14114 w14137]
              frame 0, Default {
                w14067 = 2 ("偏移量(0)")
                w14020 = ":" ("正则表达式")
                w14028 = 0.0 ("元素")
                w14047 = 256.0 ("y")
                w14052 = 256.0 ("y")
                w14064 = "-" ("正则表达式")
                n5345 = Unbundle By Name(w14060) -> ("电池包额定能量"=w14033:dbl, "电池包额定容量"=w14035:dbl, "实际容量"=w14034:dbl, "电池包额定总电压"=w14058:dbl)
                n5346 = Unbundle By Name(w14060) -> ("电池串联"=w14075:dbl, "电池并联"=w14074:dbl, "电池厂家"=w14073:string, "电池类型"=w14071:string, "电池生产日期"=w14069:string)
                n5347 = Match Pattern(string=w14069, regular expression=w14064) -> (before substring=w14068:string, after substring=w14065:string)  [unwired: 3 out]
                n5348 = Match Pattern(string=w14065, regular expression=w14064) -> (before substring=w14063:string, after substring=w14026:string)  [unwired: 3 out]
                n5349 = Match Pattern(string=w14026, regular expression=" " ("正则表达式")) -> (before substring=w14024:string, after substring=w14023:string)  [unwired: 3 out]
                n5350 = call "输入分辨率计算-EV05.vi"("1字节?"=FALSE, "数值"=w14033, "分辨率"=0.1) -> ("低字节"=w14032:dbl, "高字节1"=w14031:dbl)  [unwired: 2 in, 5 out]
                n5351 = String Subset(string=w14068, offset (0)=w14067, length (rest)=w14067) -> (substring=w14066:string)
                n5352 = call "输入分辨率计算-EV05.vi"("1字节?"=TRUE, "数值 2"=w14034, "数值"=w14035, "分辨率"=0.001) -> ("高字节 2"=w14036:dbl, "高字节1"=w14037:dbl)  [unwired: 1 in, 5 out]
                n5353 = Match Pattern(string=w14023, regular expression=w14020) -> (before substring=w14022:string, after substring=w14021:string)  [unwired: 3 out]
                n5354 = Fract/Exp String To Number(string=w14066) -> (number=w14016:dbl)  [unwired: 1 in, 3 out]
                n5355 = Fract/Exp String To Number(string=w14063) -> (number=w14015:dbl)  [unwired: 4 out]
                n5356 = Fract/Exp String To Number(string=w14024) -> (number=w14014:dbl)  [unwired: 4 out]
                n5357 = case shown="\"2\", \"盟固利\"" w14073 {
                  tunnel: [2 1] -> w14072
                  frame "2", "盟固利" {
                  }
                  frame "1", "普莱德", Default {
                  }
                }
                n5358 = case shown="\"9\", \"其他电池\"" w14071 {
                  tunnel: [2 3 4 5 6 7 8 9 1] -> w14070
                  frame "2", "锰酸锂" {
                  }
                  frame "3", "三元材料" {
                  }
                  frame "4", "铅酸" {
                  }
                  frame "5", "镍氢" {
                  }
                  frame "6", "钴酸锂" {
                  }
                  frame "7", "聚合物锂离子" {
                  }
                  frame "8", "钛酸锂" {
                  }
                  frame "9", "其他电池" {
                  }
                  frame "1", "磷酸铁锂", Default {
                  }
                }
                n5359 = Match Pattern(string=w14021, regular expression=w14020) -> (before substring=w14019:string, after substring=w14018:string)  [unwired: 3 out]
                n5360 = call "输入分辨率计算-EV05.vi"("1字节?"=FALSE, "数值"=w14058, "分辨率"=0.1) -> ("低字节"=w14029:dbl, "高字节1"=w14030:dbl)  [unwired: 2 in, 5 out]
                n5361 = Quotient & Remainder(x=w14037, y=w14052) -> (x-y*floor(x/y)=w14051:dbl, floor(x/y)=w14055:dbl)
                n5362 = Fract/Exp String To Number(string=w14022) -> (number=w14013:dbl)  [unwired: 4 out]
                n5363 = Quotient & Remainder(x=w14036, y=w14047) -> (x-y*floor(x/y)=w14043:dbl, floor(x/y)=w14044:dbl)
                n5364 = Quotient & Remainder(x=w14055, y=w14052) -> (x-y*floor(x/y)=w14050:dbl, floor(x/y)=w14054:dbl)
                n5365 = Fract/Exp String To Number(string=w14019) -> (number=w14012:dbl)  [unwired: 4 out]
                n5366 = Quotient & Remainder(x=w14044, y=w14047) -> (x-y*floor(x/y)=w14042:dbl, floor(x/y)=w14045:dbl)
                n5367 = call <vilib>:"Trim Whitespace.vi"("string"=w14018) -> ("trimmed string"=w14017:string)  [unwired: 1 in]
                n5368 = Quotient & Remainder(x=w14054, y=w14052) -> (x-y*floor(x/y)=w14049:dbl, floor(x/y)=w14053:dbl)
                n5369 = Quotient & Remainder(x=w14045, y=w14047) -> (x-y*floor(x/y)=w14041:dbl, floor(x/y)=w14046:dbl)
                n5370 = Quotient & Remainder(x=w14075, y=256.0) -> (x-y*floor(x/y)=w14077:dbl, floor(x/y)=w14078:dbl)
                n5371 = Fract/Exp String To Number(string=w14017) -> (number=w14011:dbl)  [unwired: 4 out]
                n5372 = Quotient & Remainder(x=w14053, y=w14052) -> (x-y*floor(x/y)=w14048:dbl)  [unwired: 1 out]
                n5373 = Quotient & Remainder(x=w14046, y=w14047) -> (x-y*floor(x/y)=w14040:dbl)  [unwired: 1 out]
                n5374 = Build Array(w14031, w14032, w14048, w14049, w14050, w14051, w14040, w14041, w14042, w14043, w14030, w14029, w14028, w14028, w14028, w14016, w14015, w14014, w14013, w14012, w14011) -> (w14027:dbl[])
                n5375 = Build Array(w14078, w14077, w14074, w14072, w14070) -> (w14076:dbl[])
                n5376 = Insert Into Array(array=w14076, new element=w14027) -> (w14059:dbl[])  [unwired: 1 in]
              }
              frame 1 {
                w14095 = 256.0 ("y")
                n5377 = Unbundle By Name(w14104) -> ("电池包组号"=w14103:string)
                n5378 = Match Pattern(string=w14103, regular expression="-" ("正则表达式")) -> (before substring=w14101:string, after substring=w14100:string)  [unwired: 3 out]
                n5379 = Fract/Exp String To Number(string=w14101) -> (number=w14099:dbl)  [unwired: 1 in, 3 out]
                n5380 = Fract/Exp String To Number(string=w14100) -> (number=w14096:dbl)  [unwired: 4 out]
                n5381 = Quotient & Remainder(x=w14096, y=w14095) -> (x-y*floor(x/y)=w14093:dbl, floor(x/y)=w14094:dbl)
                n5382 = Quotient & Remainder(x=w14099, y=w14095) -> (x-y*floor(x/y)=w14097:dbl, floor(x/y)=w14098:dbl)
                n5383 = Build Array(w14098, w14097, w14094, w14093) -> (w14105:dbl[])
              }
              frame 2 {
                w14122 = 256.0 ("y")
                w14127 = 256.0 ("y")
                n5384 = Unbundle By Name(w14114) -> ("累计充电总安时"=w14111:dbl, "累计放电总安时"=w14110:dbl)
                n5385 = call "输入分辨率计算-EV05.vi"("1字节?"=TRUE, "数值 2"=w14110, "数值"=w14111, "分辨率"=0.001) -> ("高字节 2"=w14108:dbl, "高字节1"=w14109:dbl)  [unwired: 1 in, 5 out]
                n5386 = Quotient & Remainder(x=w14109, y=w14127) -> (x-y*floor(x/y)=w14126:dbl, floor(x/y)=w14130:dbl)
                n5387 = Quotient & Remainder(x=w14108, y=w14122) -> (x-y*floor(x/y)=w14118:dbl, floor(x/y)=w14119:dbl)
                n5388 = Quotient & Remainder(x=w14130, y=w14127) -> (x-y*floor(x/y)=w14125:dbl, floor(x/y)=w14129:dbl)
                n5389 = Quotient & Remainder(x=w14119, y=w14122) -> (x-y*floor(x/y)=w14117:dbl, floor(x/y)=w14120:dbl)
                n5390 = Quotient & Remainder(x=w14129, y=w14127) -> (x-y*floor(x/y)=w14124:dbl, floor(x/y)=w14128:dbl)
                n5391 = Quotient & Remainder(x=w14120, y=w14122) -> (x-y*floor(x/y)=w14116:dbl, floor(x/y)=w14121:dbl)
                n5392 = Quotient & Remainder(x=w14128, y=w14127) -> (x-y*floor(x/y)=w14123:dbl)  [unwired: 1 out]
                n5393 = Quotient & Remainder(x=w14121, y=w14122) -> (x-y*floor(x/y)=w14115:dbl)  [unwired: 1 out]
                n5394 = Build Array(w14123, w14124, w14125, w14126, w14115, w14116, w14117, w14118) -> (w14131:dbl[])
              }
              frame 3 {
                w14142 = 256.0 ("y")
                n5395 = Unbundle By Name(w14137) -> ("电池放空次数"=w14136:dbl, "电池充满次数"=w14135:dbl, "电池充电次数"=w14134:dbl)
                n5396 = Quotient & Remainder(x=w14136, y=w14142) -> (x-y*floor(x/y)=w14144:dbl, floor(x/y)=w14145:dbl)
                n5397 = Quotient & Remainder(x=w14135, y=w14142) -> (x-y*floor(x/y)=w14140:dbl, floor(x/y)=w14141:dbl)
                n5398 = Quotient & Remainder(x=w14134, y=w14142) -> (x-y*floor(x/y)=w14138:dbl, floor(x/y)=w14139:dbl)
                n5399 = Build Array(w14145, w14144, w14141, w14140, w14139, w14138) -> (w14143:dbl[])
              }
            }
          }
        }
        frame "电池信息" {
          n5400 = Unbundle By Name(w14151) -> ("电池信息"=w14152:refnum<vi>)
          n5401 = property class="Clust (严格)"(reference=w14152) -> ("Value"=w14150:T7)  [unwired: 1 in, 2 out]
          n5402 = for {
            N: 4 -> [_]
            tunnel: [w14163] -> w14156 mode=indexing
            tunnel: [w14162] -> w14155 mode=indexing
            tunnel: [w14160] -> w14153 mode=indexing
            tunnel: w14150 -> [w14159]
            tunnel: [w14158] -> w14148 mode=indexing
            i -> [w14161]
            n5403 = case shown="1" w14161 {
              tunnel: [30 ("单个参数补充") 4 ("单个参数补充") 8 ("单个参数补充") 6 ("单个参数补充")] -> w14163
              tunnel: [1 ("命令序号") 2 ("命令序号") 3 ("命令序号") 4 ("命令序号")] -> w14162
              tunnel: [w14213 w14247 w14287 w14300] -> w14160
              tunnel: w14159 -> [w14214 w14248 w14270 w14294]
              tunnel: ["电池组信息1" "电池包组号" "充放电安时" "电池充放电次数"] -> w14158
              frame 0, Default {
                w14221 = 2 ("偏移量(0)")
                w14173 = ":" ("正则表达式")
                w14181 = 0.0 ("元素")
                w14200 = 256.0 ("y")
                w14205 = 256.0 ("y")
                w14218 = "-" ("正则表达式")
                n5404 = Unbundle By Name(w14214) -> ("电池包额定能量"=w14186:dbl, "电池包额定容量"=w14188:dbl, "实际容量"=w14187:dbl, "电池包额定总电压"=w14211:dbl)
                n5405 = Unbundle By Name(w14214) -> ("电池串联"=w14229:dbl, "电池并联"=w14228:dbl, "电池厂家"=w14227:string, "电池类型"=w14225:string, "电池生产日期"=w14223:string)
                n5406 = Match Pattern(string=w14223, regular expression=w14218) -> (before substring=w14222:string, after substring=w14219:string)  [unwired: 3 out]
                n5407 = Match Pattern(string=w14219, regular expression=w14218) -> (before substring=w14217:string, after substring=w14179:string)  [unwired: 3 out]
                n5408 = Match Pattern(string=w14179, regular expression=" " ("正则表达式")) -> (before substring=w14177:string, after substring=w14176:string)  [unwired: 3 out]
                n5409 = call "输入分辨率计算-EV05.vi"("1字节?"=FALSE, "数值"=w14186, "分辨率"=0.1) -> ("低字节"=w14185:dbl, "高字节1"=w14184:dbl)  [unwired: 2 in, 5 out]
                n5410 = String Subset(string=w14222, offset (0)=w14221, length (rest)=w14221) -> (substring=w14220:string)
                n5411 = call "输入分辨率计算-EV05.vi"("1字节?"=TRUE, "数值 2"=w14187, "数值"=w14188, "分辨率"=0.001) -> ("高字节 2"=w14189:dbl, "高字节1"=w14190:dbl)  [unwired: 1 in, 5 out]
                n5412 = Match Pattern(string=w14176, regular expression=w14173) -> (before substring=w14175:string, after substring=w14174:string)  [unwired: 3 out]
                n5413 = Fract/Exp String To Number(string=w14220) -> (number=w14169:dbl)  [unwired: 1 in, 3 out]
                n5414 = Fract/Exp String To Number(string=w14217) -> (number=w14168:dbl)  [unwired: 4 out]
                n5415 = Fract/Exp String To Number(string=w14177) -> (number=w14167:dbl)  [unwired: 4 out]
                n5416 = case shown="\"2\", \"盟固利\"" w14227 {
                  tunnel: [2 1] -> w14226
                  frame "2", "盟固利" {
                  }
                  frame "1", "普莱德", Default {
                  }
                }
                n5417 = case shown="\"9\", \"其他电池\"" w14225 {
                  tunnel: [2 3 4 5 6 7 8 9 1] -> w14224
                  frame "2", "锰酸锂" {
                  }
                  frame "3", "三元材料" {
                  }
                  frame "4", "铅酸" {
                  }
                  frame "5", "镍氢" {
                  }
                  frame "6", "钴酸锂" {
                  }
                  frame "7", "聚合物锂离子" {
                  }
